vi "to table.vi"(8 "error in (no error)":errorcluster, 10 "variant":variant, 11 "configuration in":refnum<class "NISE_CEF_serializable configuration.lvclass">) -> (0 "error out":errorcluster, 2 "table":string[][](array[string]), 3 "configuration out":refnum<class "NISE_CEF_serializable configuration.lvclass">)   [LabVIEW 2013, in "NISE_CEF_serializable configuration.lvclass"]
uses:
  NISE_CEF_serializable configuration.lvclass
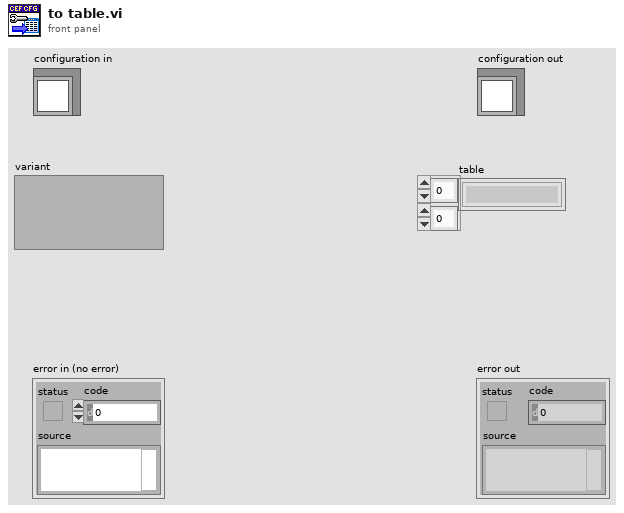
[diagram p1: front panel]
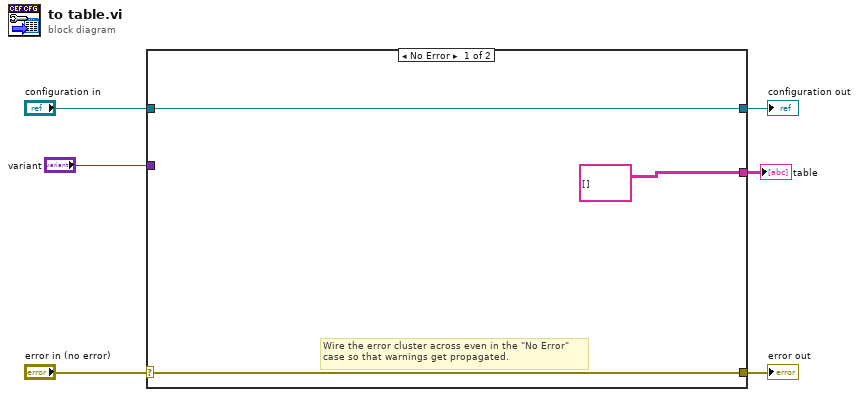
[diagram p0: block diagram]
diagram:
  n1 = case shown="No Error" "error in (no error)" {
    selector: "error in (no error)" -> [w8 w11]
    tunnel: [w8 w11] -> w5
    tunnel: [w9 w10] -> w3
    tunnel: "configuration in" -> [w9 w10]
    tunnel: "variant" -> [_ _]
    tunnel: [string[][] [] ("table") _] -> w1
    frame No Error {
      # "Wire the error cluster across even in the \"No Error\"\ncase so that warnings get propagated."
    }
    frame Error {
    }
  }
  "error out" <- w5
  "configuration out" <- w3
  "table" <- w1
